vi "contours2ROI.vi"(11 "Segment Information":T2(array[cluster])) -> (0 "ROI origin":T1(array[cluster]), 3 "ROI":T1(array[cluster]))   [LabVIEW 2017]
panel:
  in  "again":bool
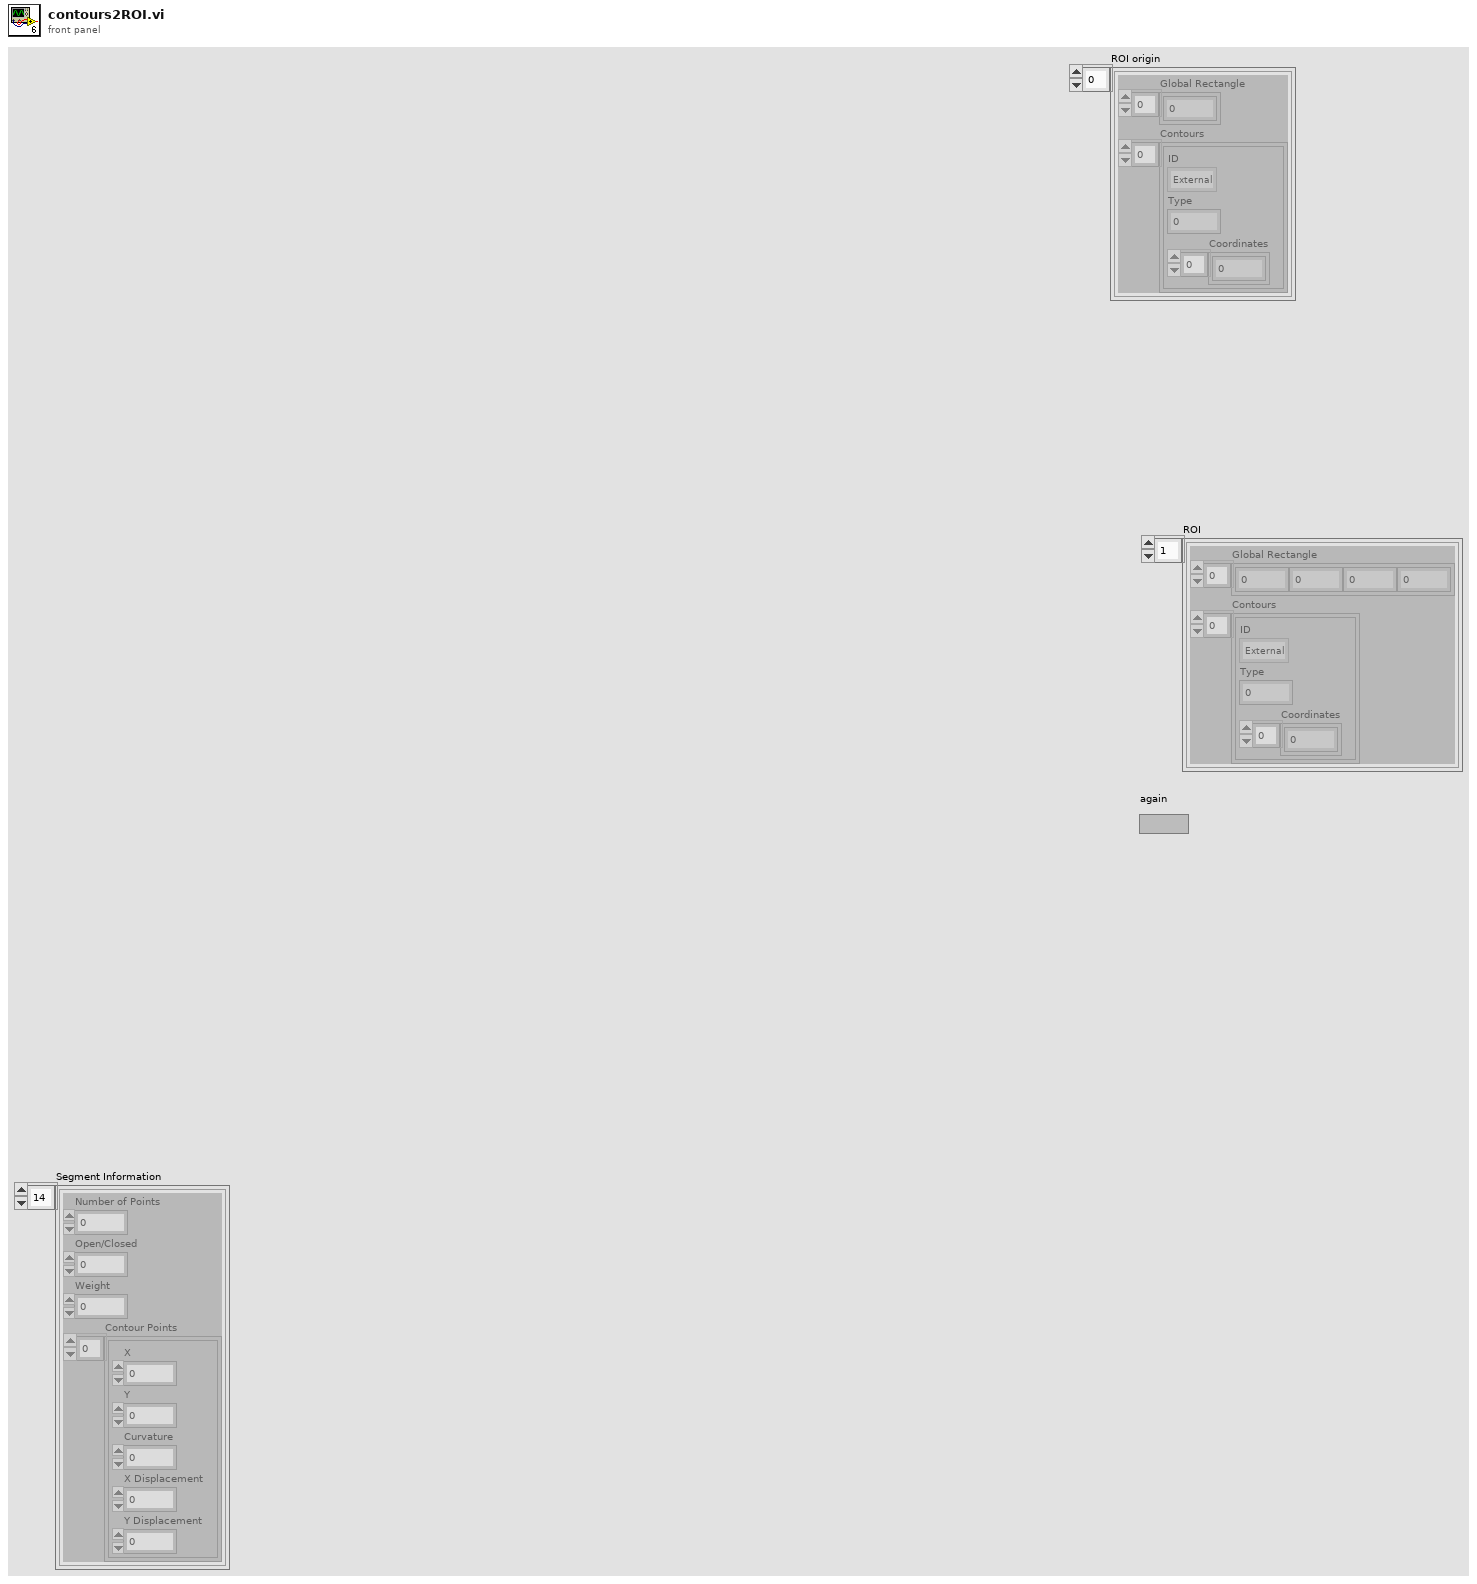
[diagram p1: front panel]
types:
  T1 = cluster{"Global Rectangle":dbl[], "Contours":cluster{"ID":enum32{"External", "Internal"}, "Type":u32, "Coordinates":i32[]}[]}[]
  T2 = cluster{"Number of Points":i32, "Open/Closed":i32, "Weight":dbl, "Contour Points":cluster{"X":dbl, "Y":dbl, "Curvature":dbl, "X Displacement":dbl, "Y Displacement":dbl}[]}[]
  T3 = cluster{"X":dbl, "Y":dbl, "Curvature":dbl, "X Displacement":dbl, "Y Displacement":dbl}[]
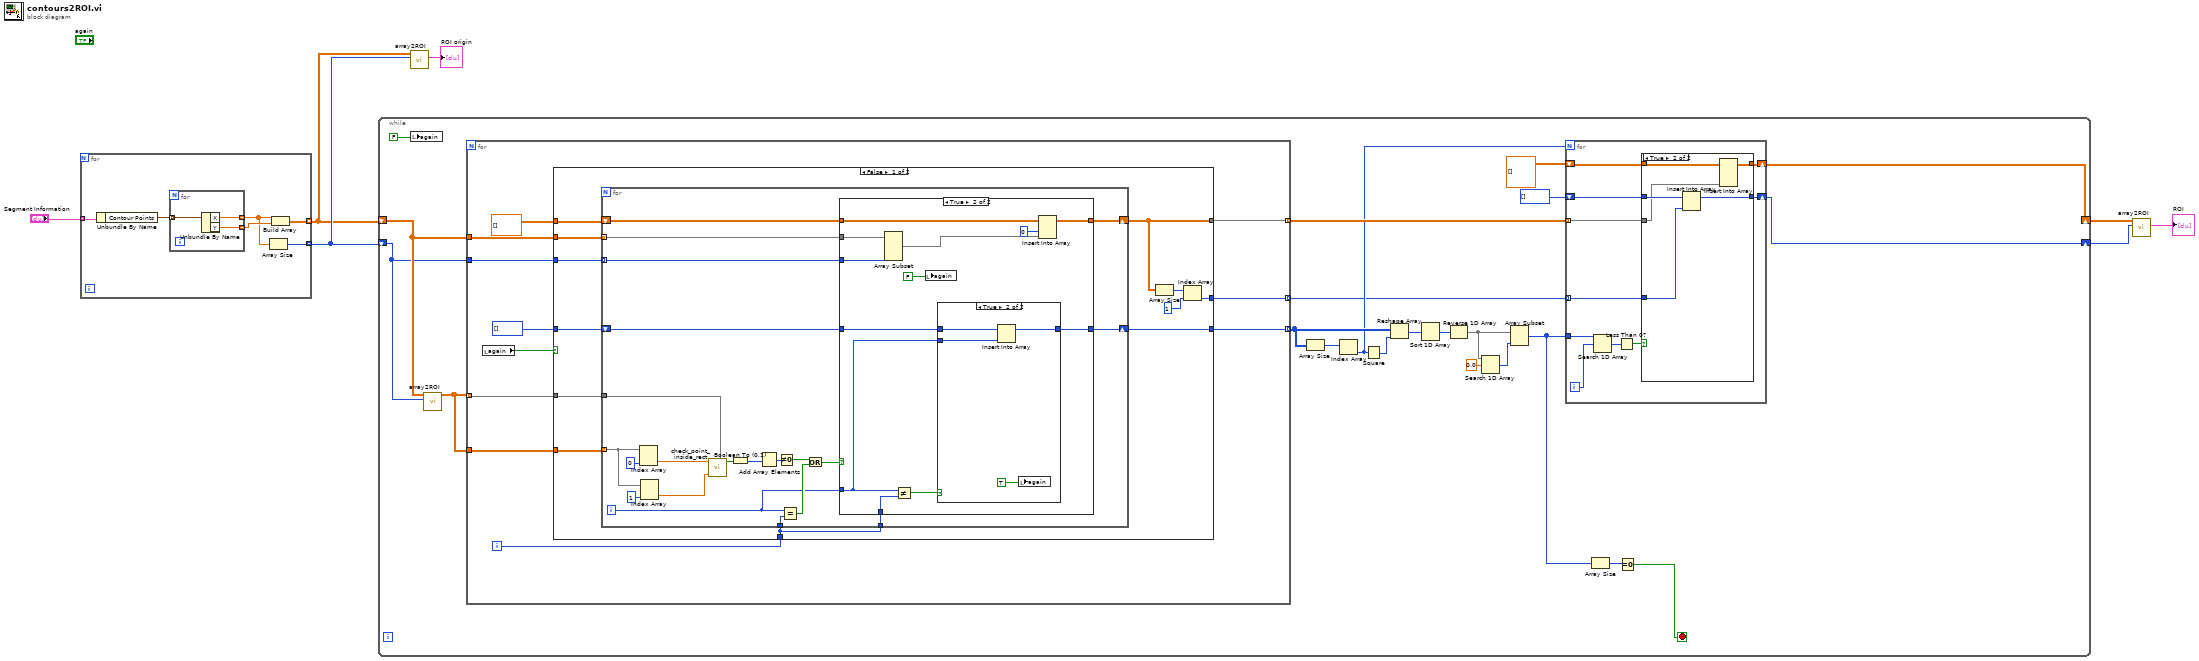
[diagram p0: block diagram]
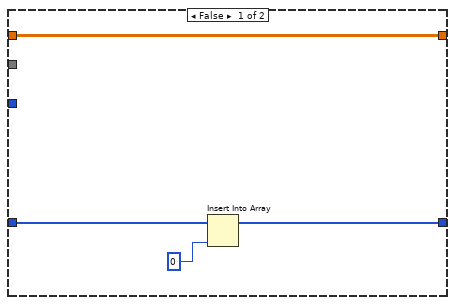
[diagram p3: hidden frame]
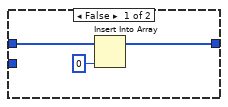
[diagram p4: hidden frame]
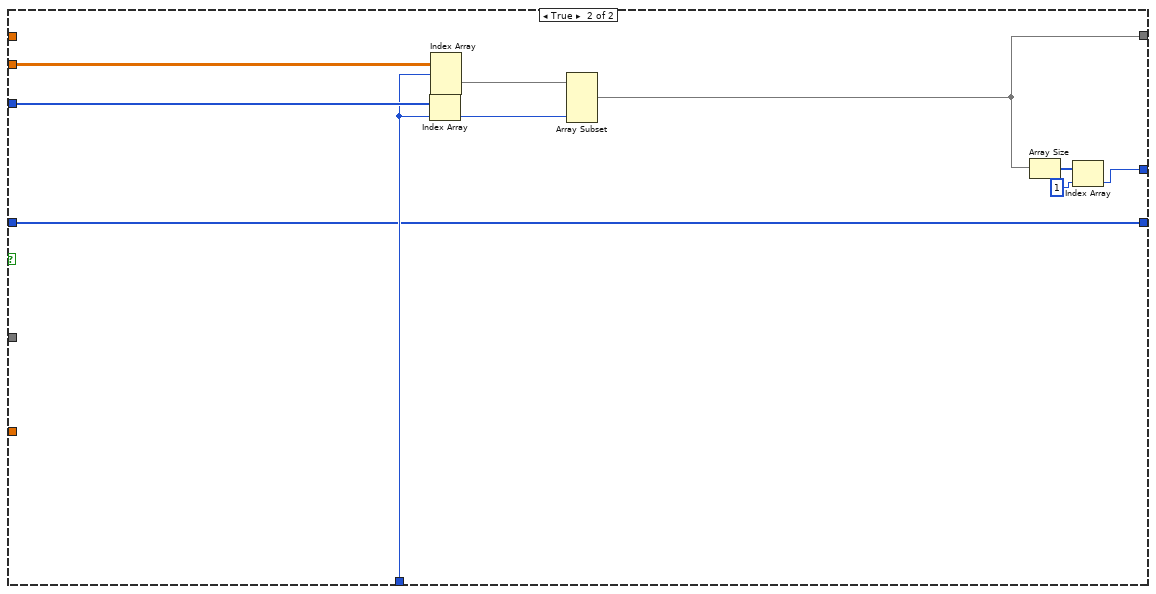
[diagram p5: hidden frame]
diagram:
  n1 = for {
    tunnel: "Segment Information" -> [w13] mode=indexing
    tunnel: [w10] -> w1 mode=indexing
    tunnel: [w8] -> w3 mode=indexing
    n2 = Unbundle By Name(w13) -> ("Contour Points"=w12:T3)
    n3 = for {
      tunnel: w12 -> [w16] mode=indexing
      tunnel: [w15] -> w9 mode=indexing
      tunnel: [w14] -> w11 mode=indexing
      n4 = Unbundle By Name(w16) -> ("X"=w15:dbl, "Y"=w14:dbl)
    }
    n5 = Array Size(array=w9) -> (size(s)=w8:i32)
    n6 = Build Array(w9, w11) -> (w10:dbl[][])
  }
  n7 = while {
    shift-right: [w26] -> w4
    shift-left: w1 -> [w38]
    shift-right: [w22] -> w6
    shift-left: w3 -> [w19]
    stop <- w20 stop-if-true
    n8 = local write "again"(FALSE) -> ()
    n9 = call "array2ROI.vi"("length"=w19, "array"=w38) -> ("corner"=w18:dbl[][][])  [unwired: 8 in, 1 out]
    n10 = for {
      tunnel: w38 -> [w66]
      tunnel: w19 -> [w65]
      tunnel: w18 -> [w57] mode=indexing
      tunnel: w18 -> [w67]
      tunnel: [w63] -> w29 mode=indexing
      tunnel: [w62] -> w23 mode=indexing
      tunnel: [w59] -> w36 mode=indexing
      i -> [w58]
      n11 = local read "again"() -> (w60:bool)
      n12 = case shown="False" w60 {
        tunnel: w67 -> [w79 _]
        tunnel: w57 -> [w78 _]
        tunnel: w66 -> [w77 w131]
        tunnel: w65 -> [w76 w129]
        tunnel: dbl[][] [] -> [w75 _]
        tunnel: [w74 w126] -> w63
        tunnel: [w73 w132] -> w62
        tunnel: w58 -> [w71 w128]
        tunnel: i32[] [] -> [w70 w125]
        tunnel: [w69 w125] -> w59
        frame False {
          n13 = for {
            tunnel: w79 -> [w94] mode=indexing
            tunnel: w78 -> [w92]
            tunnel: w71 -> [w91]
            tunnel: w77 -> [w85] mode=indexing
            shift-right: [w86] -> w74
            shift-left: w75 -> [w87]
            tunnel: w76 -> [w84] mode=indexing
            tunnel: w71 -> [w83]
            shift-right: [w80] -> w69
            shift-left: w70 -> [w81]
            i -> [w82]
            n14 = Index Array(array=w94, index (col)=0 ("disabled index (col)")) -> (element=w98:dbl[])  [unwired: 1 in]
            n15 = Index Array(array=w94, index (col)=1) -> (element=w97:dbl[])  [unwired: 1 in]
            n16 = call "check_point_inside_rect.vi"("rectangle corner"=w92, "Y"=w97, "X"=w98) -> ("result"=w93:bool[])  [unwired: 8 in]
            n17 = Boolean To (0,1)(Boolean=w93) -> (0, 1=w96:i16[])
            n18 = Add Array Elements(numeric array=w96) -> (sum=w95:i16)
            n19 = Not Equal To 0?(x=w95) -> (x != 0?=w89:bool)
            n20 = Equal?(x=w82, y=w91) -> (x = y?=w90:bool)
            n21 = Or(x=w89, y=w90) -> (x .or. y?=w88:bool)
            n22 = case shown="True" w88 {
              tunnel: w87 -> [w104 w116]
              tunnel: [w104 w115] -> w86
              tunnel: w85 -> [_ w114]
              tunnel: w84 -> [_ w113]
              tunnel: w83 -> [_ w111]
              tunnel: w82 -> [_ w106]
              tunnel: w81 -> [w102 w109]
              tunnel: [w101 w108] -> w80
              frame False {
                n23 = Insert Into Array "Insert Into Array"(array=w102, new element=0) -> (w101:i32[])  [unwired: 1 in]
              }
              frame True {
                n24 = Array Subset "Array Subset"(array=w114, length (col)=w113) -> (w112:dbl[][])  [unwired: 3 in]
                n25 = Not Equal?(x=w106, y=w111) -> (x != y?=w110:bool)
                n26 = local write "again"(FALSE) -> ()
                n27 = case shown="True" w110 {
                  tunnel: w109 -> [w119 w123]
                  tunnel: [w118 w122] -> w108
                  tunnel: w106 -> [_ w120]
                  frame False {
                    n28 = Insert Into Array(array=w119, new element=0 ("new element/subarray")) -> (w118:i32[])  [unwired: 1 in]
                  }
                  frame True {
                    n29 = Insert Into Array "Insert Into Array"(array=w123, new element=w120) -> (w122:i32[])  [unwired: 1 in]
                    n30 = local write "again"(TRUE) -> ()
                  }
                }
                n31 = Insert Into Array "Insert Into Array"(array=w116, index (col)=0 ("disabled index (col)"), new element=w112) -> (w115:dbl[][])  [unwired: 1 in]
              }
            }
          }
          n32 = Array Size(array=w74) -> (size(s)=w68:i32[])
          n33 = Index Array(array=w68, index=1) -> (element=w73:i32)
        }
        frame True {
          n34 = Index Array(array=w129, index=w128) -> (element=w127:i32)
          n35 = Index Array "Index Array"(array=w131, index (dim 0)=w128) -> (element=w130:dbl[][])  [unwired: 2 in]
          n36 = Array Subset "Array Subset"(array=w130, length (col)=w127) -> (w126:dbl[][])  [unwired: 3 in]
          n37 = Array Size(array=w126) -> (size(s)=w124:i32[])
          n38 = Index Array(array=w124, index=1) -> (element=w132:i32)
        }
      }
    }
    n39 = Array Size(array=w36) -> (size(s)=w34:i32[])
    n40 = Index Array(array=w34) -> (element=w28:i32)  [unwired: 1 in]
    n41 = Square(x=w28) -> (x^2=w33:i32)
    n42 = Reshape Array(w36, w33) -> (w35:i32[])
    n43 = Sort 1D Array(array=w35) -> (sorted array=w32:i32[])
    n44 = Reverse 1D Array(array=w32) -> (reversed array=w24:i32[])
    n45 = Search 1D Array(1D array=w24, element=0.0) -> (index of element=w30:i32)  [unwired: 1 in]
    n46 = Array Subset(array=w24, length=w30) -> (w21:i32[])  [unwired: 1 in]
    n47 = for {
      N: w28 -> [_]
      tunnel: w21 -> [w48]
      tunnel: w29 -> [w42] mode=indexing
      tunnel: w23 -> [w41] mode=indexing
      shift-right: [w44] -> w26
      shift-left: dbl[][][] [] -> [w46]
      shift-right: [w43] -> w22
      shift-left: i32[] [] -> [w45]
      i -> [w47]
      n48 = Search 1D Array(1D array=w48, element=w47) -> (index of element=w40:i32)  [unwired: 1 in]
      n49 = Less Than 0?(x=w40) -> (x < 0?=w39:bool)
      n50 = case shown="True" w39 {
        tunnel: w46 -> [w50 w56]
        tunnel: w45 -> [w49 w54]
        tunnel: [w50 w55] -> w44
        tunnel: [w49 w52] -> w43
        tunnel: w42 -> [_ w51]
        tunnel: w41 -> [_ w53]
        frame False {
        }
        frame True {
          n51 = Insert Into Array "Insert Into Array"(array=w54, new element=w53) -> (w52:i32[])  [unwired: 1 in]
          n52 = Insert Into Array(array=w56, new element=w51) -> (w55:dbl[][][])  [unwired: 3 in]
        }
      }
    }
    n53 = Array Size(array=w21) -> (size(s)=w17:i32)
    n54 = Equal To 0?(x=w17) -> (x = 0?=w20:bool)
  }
  n55 = call "array2ROI.vi"("length"=w3, "array"=w1) -> ("ROI"=→"ROI origin":T1)  [unwired: 8 in, 1 out]
  n56 = call "array2ROI.vi"("length"=w6, "array"=w4) -> ("ROI"=→"ROI":T1)  [unwired: 8 in, 1 out]
